vi "freqAndNote.vi"(10 "dt Original":dbl, 11 "Frequency In":dbl) -> (2 "output dt":dbl, 3 "Frequency Off":dbl, 4 "Note Frequency":dbl, 6 "Note Closest To":string)   [LabVIEW 2012]
uses:
  <vilib>/Utility/file.llb/Read From Spreadsheet File (string).vi
panel:
  # "This will pull out frequency difference and note and generate a dt to change frequency of signal.\nFirst generate note cluster array..."
  # "still fixing dt part I think it works though"
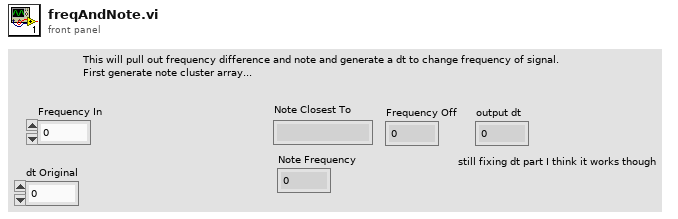
[diagram p1: front panel]
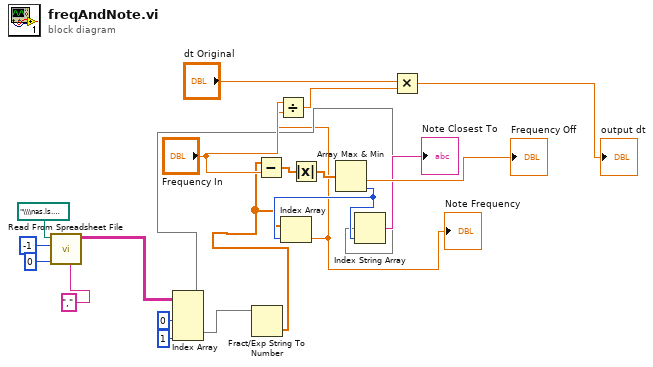
[diagram p0: block diagram]
diagram:
  n1 = call-poly <vilib>:"Read From Spreadsheet File.vi"("delimiter (\\t)"=",", "max characters/row  (no limit:0)"=0, "number of rows (all:-1)"=-1, "file path (dialog if empty)"=path "\\\\nas.ls.berkeley.edu\\111lab/Student-Redirect$/joshualevy44/Desktop/111A Final/Other/scales.csv") -> ("all rows"=w9:string[][])  [unwired: 3 in, 4 out]
  n2 = Index Array(array=w9, index (col) #1=0 ("disabled index (col)"), index (col) #2=1 ("index (col)")) -> (element #1=w4:string[], element #2=w6:string[])  [unwired: 2 in]
  n3 = Fract/Exp String To Number(string=w6) -> (number=w5:dbl[])  [unwired: 3 in, 1 out]
  n4 = Subtract(x=w5, y="Frequency In") -> (x-y=w20:dbl[])
  n5 = Absolute Value(x=w20) -> (abs(x)=w19:dbl[])
  n6 = Array Max & Min(array=w19) -> (min value=→"Frequency Off":dbl, min index (indices)=w15:i32)  [unwired: 2 out]
  n7 = Index Array(array=w5, index=w15) -> (element=w2:dbl)
  "Note Frequency" <- w2
  n8 = Divide(x="Frequency In", y=w2) -> (x/y=w13:dbl)
  n9 = Index String Array(1:w15, 2:w4) -> (0:→"Note Closest To":string)  [unwired: 1 in]
  n10 = Multiply(x="dt Original", y=w13) -> (x*y=→"output dt":dbl)
